vi "MasterAcquisitionFile_IOS_Test.vi"() -> ()   [LabVIEW 2020]
uses:
  <vilib>/vision/driver/IMAQdx.llb/IMAQdx Camera Control Mode.ctl
  <vilib>/vision/driver/IMAQdx.llb/IMAQdx Acquisition Mode.ctl
  <vilib>/userDefined/High Color/IMAQdx.ctl
  <vilib>/vision/driver/IMAQdx.llb/IMAQdx Buffer Number Mode.ctl
  <vilib>/DAQmx/write.llb/DAQmx Write (Digital 1D Wfm NChan NSamp).vi
  <vilib>/DAQmx/read.llb/DAQmx Read (Analog 1D Wfm NChan NSamp).vi
  <vilib>/Waveform/DWDTOps.llb/DWDT Digital to Boolean Array.vi
  <vilib>/DAQmx/create/channels.llb/DAQmx Create Channel (CO-Pulse Generation-Frequency).vi
  <vilib>/DAQmx/configure/timing.llb/DAQmx Timing (Implicit).vi
  <vilib>/DAQmx/create/channels.llb/DAQmx Create Channel (AI-Voltage-Basic).vi
  <vilib>/DAQmx/configure/timing.llb/DAQmx Timing (Sample Clock).vi
  <vilib>/DAQmx/configure/trigger.llb/DAQmx Start Trigger (Digital Edge).vi
  <vilib>/DAQmx/create/channels.llb/DAQmx Create Channel (DO-Digital Output).vi
  <vilib>/Waveform/DWDTOps.llb/DWDT Boolean Array to Digital.vi
  <vilib>/Waveform/DWDTOps.llb/DWDT Uncompress Digital.vi
  <vilib>/DAQmx/miscellaneous.llb/DAQmx Fill In Error Info.vi
  <vilib>/vision/driver/NI_Vision_Acquisition_Software.lvlib
  <resource>/objmgr/imaqdx.rc
  <resource>/objmgr/daqmx.rc
panel:
  out "LED":bool
  out "Auditory":bool
  out "RPad":bool
  out "LPad":bool
  out "Finished":bool
  in  "Generate Stimuli":bool=TRUE
  in  "Sol Stim Parameters":cluster{"Fs":dbl, "Samples":dbl}
  in  "LED Stim Parameters":cluster{"Fs":dbl, "Samples":dbl}
  in  "Sol Duty Cycle (%)":dbl=10.0
  in  "Sol Freq":dbl=1.0
  in  "Sol Dur (s)":dbl=1.0
  in  "LED Duty Cycle (%)":dbl=10.0
  in  "LED Freq":dbl=10.0
  in  "LED Dur (s)":dbl=2.0
  out "Stimulus Order":digitalwaveform[](graph)=[{"t0"=timestamp(0 s since 1904-01-01), "dt"=5e-05, "Y"={"transitions"=[], "data"=array18001000x1[18001000 elements]}}, {"t0"=timestamp(0 s since 1904-01-01), "dt"=5e-05, "Y"={"transitions"=[], "data"=array18001000x1[18001000 elements]}}, {"t0"=timestamp(0 s since 1904-01-01), "dt"=5e-05, "Y"={"transitions"=[], "data"=array18001000x1[18001000 elements]}}, {"t0"=timestamp(0 s since 1904-01-01), "dt"=5e-05, "Y"={"transitions"=[], "data"=array18001000x1[18001000 elements]}}]
  out "Solenoid Stim":digitalwaveform(graph)={"t0"=timestamp(0 s since 1904-01-01), "dt"=5e-05, "Y"={"transitions"=[], "data"=array20000x1[20000 elements]}}
  in  "Trial Offset (s)":dbl=15.0
  in  "Interstim (s)":dbl=30.0
  in  "Right Pad":dbl=1.0
  in  "Left Pad":dbl=1.0
  in  "Auditory":dbl=1.0
  in  "LED":dbl
  out "?":T1(plugin-control)
  out "?":T1(plugin-control)
  out "?":T1(plugin-control)
  out "?":T1(plugin-control)
  in  "stop":bool
  out "CBV Cam":bool=TRUE
  out "Pupil Cam":bool=TRUE
  out "Whisk Cam":bool=TRUE
  out "Web Cam":bool=TRUE
  out "Analog":bool=TRUE
  out "Web Cam Fs":dbl(knob)=30.0 scale=0.0..200.0
  out "CBV Cam Fs":dbl(knob)=30.019685039370078 scale=0.0..200.0
  out "Whisk Cam Fs":dbl(knob)=149.92503748125938 scale=0.0..200.0
  out "Last Whisk\nBuffer 2":u32=160
  out "Pupil Cam Fs":dbl(knob)=30.0 scale=0.0..200.0
  out "Dropped 2":u32(slide) caption="Pupil Cam" scale=0.0..99.0
  in  "Exposure Time (microsec)":string="10000"
  out "Dev1 Samples":i32=107434
  in  "Dev1 Analog Channels":string[](array[string])=["Cortical_LH", "Force_Sensor", "LPadSol", "RPadSol", "AudSol", "Hippocampus", "EMG", "Cortical_RH", "OptoLED"]
  in  "Analog Acquisition":cluster{"Analog Fs":u16}={"Analog Fs"=20000} {"Analog Fs" format="%0.0f"}
  in  "Sampling Rates":T2={"CBV Cam Fs"=30, "Whisk Cam Fs"=150, "Web Cam Fs"=15, "Pupil Cam Fs"=30}
  out "Notes Size":i32=8
  out "Notes Reversed":string[](array[string])=["Experimenter", "Animal ID", "Hemisphere", "Solenoid PSI", "Isoflurane time", "Session ID", "Amplifier Gain", "LED power (mW)"]
  out "Notes Array":string[](array[string])=["LED power (mW)", "Amplifier Gain", "Session ID", "Isoflurane time", "Solenoid PSI", "Hemisphere", "Animal ID", "Experimenter"]
  in  "Notes:":T3={"Experimenter"="Kevin", "Animal ID"="T220", "Hemisphere"="Both", "Solenoid PSI"="10", "Isoflurane time"="1000", "Session ID"="Imaging Session One", "Amplifier Gain"="10000", "LED power (mW)"="10"}
  in  "Target Path":path=path "D:/T220/Imaging Session One - 17 May 2021" caption="Final Save Location"
  out "Dropped":u32(slide) caption="Whisk Cam" scale=0.0..999.0
  out "Filename":string="210517_10_15_02"
  out "CBV Camera":bool
  out "Time Elapsed (Min)":cluster{dbl, dbl}(slide)={15.0, 0.08920117000000001} scale=0.0..15.0 scale format="%#_2g"
  in  "Time (min)":dbl(knob)=15.0 min=0.5 max=20.0 step=0.5 scale=0.0..20.0 scale format="%#_2g"
  in  "Temp Path":path=path "D:/LabVIEW Streamed Data" caption="Temporary Path for Streamed Data"
  out "Last CBV\nBuffer":i32=160
  out "Last Whisk\nBuffer":u32=804
  # "Dropped Frames"
  # "Stimuli"
  # "LPAD"
  # "RPAD"
  # "AUD"
  # "LED"
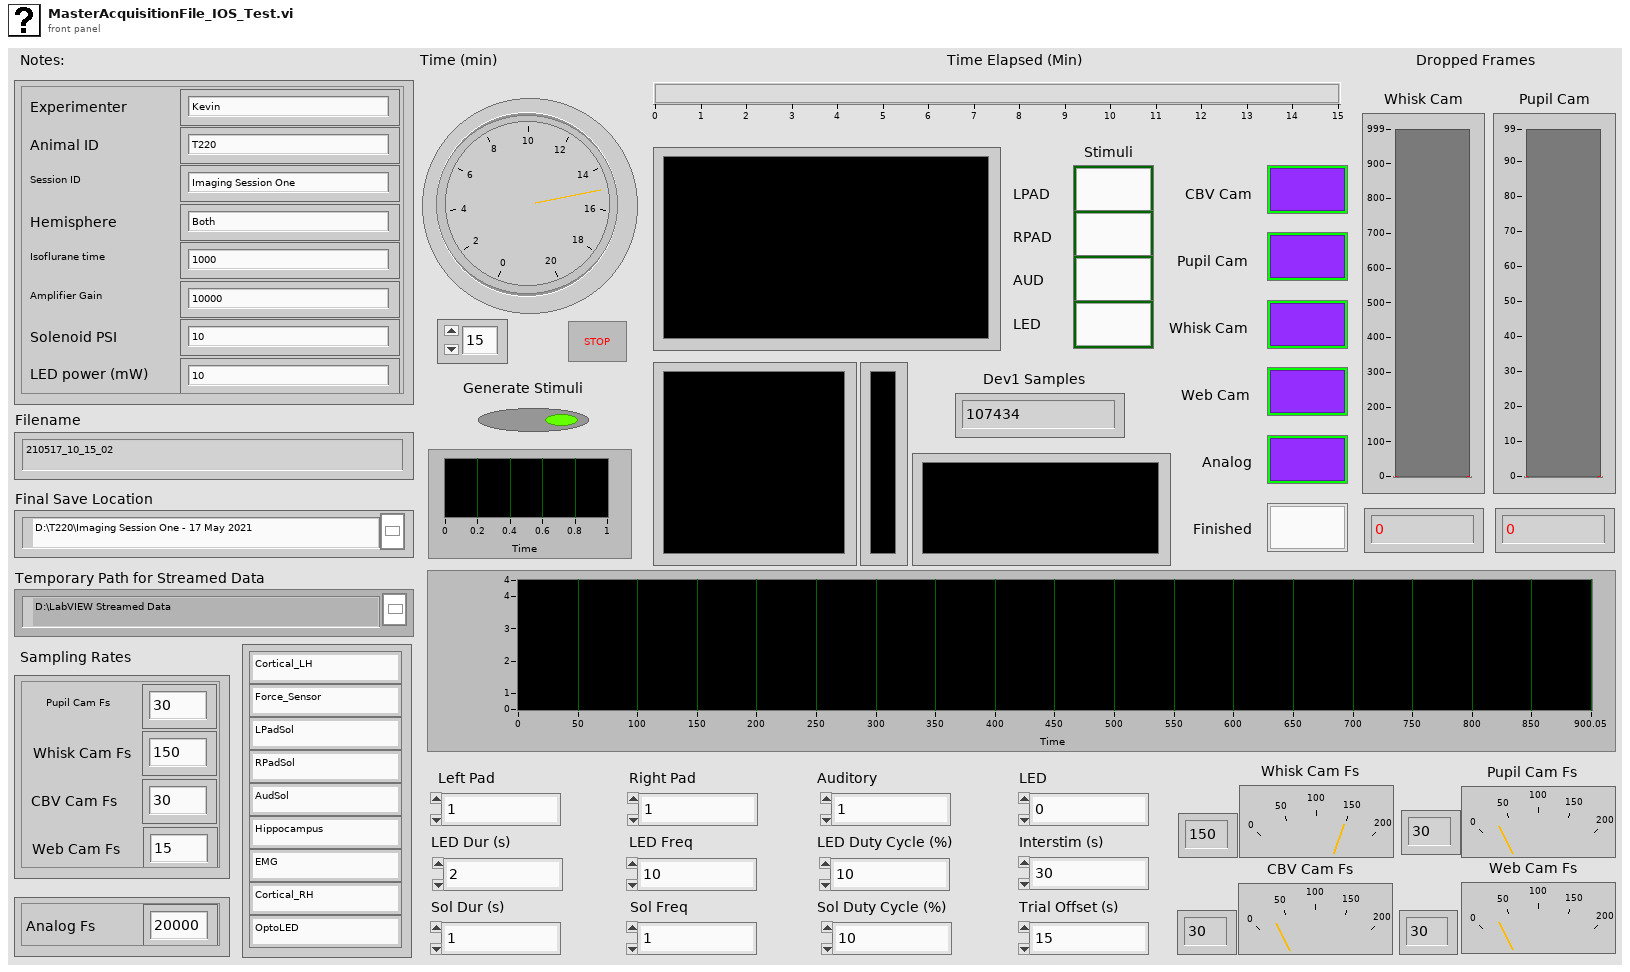
[diagram p1: front panel]
types:
  T1 = typedef "IMAQ Image.ctl" = refnum<image>
  T2 = cluster{"CBV Cam Fs":u16, "Whisk Cam Fs":u16, "Web Cam Fs":u16, "Pupil Cam Fs":u16}
  T3 = cluster{"Experimenter":string, "Animal ID":string, "Hemisphere":string, "Solenoid PSI":string, "Isoflurane time":string, "Session ID":string, "Amplifier Gain":string, "LED power (mW)":string}
  T4 = typedef "IMAQdx.ctl" = refnum<k21>
  T5 = enum16{"open", "replace", "create", "open or create", "replace or create", "replace or create with confirmation"}
  T6 = typedef "Image Type" = u32
  T7 = typedef "NI_Vision_Acquisition_Software.lvlib/IMAQdx Acquisition Mode.ctl" = enum32{"One Shot", "Continuous"}
  T8 = typedef "NI_Vision_Acquisition_Software.lvlib/IMAQdx Camera Control Mode.ctl" = enum32{"Controller", "Listener"}
  T9 = enum16{"open", "open or create", "create or replace", "create", "open (read-only)"}
  T10 = typedef "IMAQ AVI2 Refnum.ctl" = refnum<k20>
  T11 = enum16{"big-endian, network order", "native, host order", "little-endian"}
  T12 = typedef "NI_Vision_Acquisition_Software.lvlib/IMAQdx Buffer Number Mode.ctl" = enum32{"Next", "Last", "Buffer Number", "Every", "Last New"}
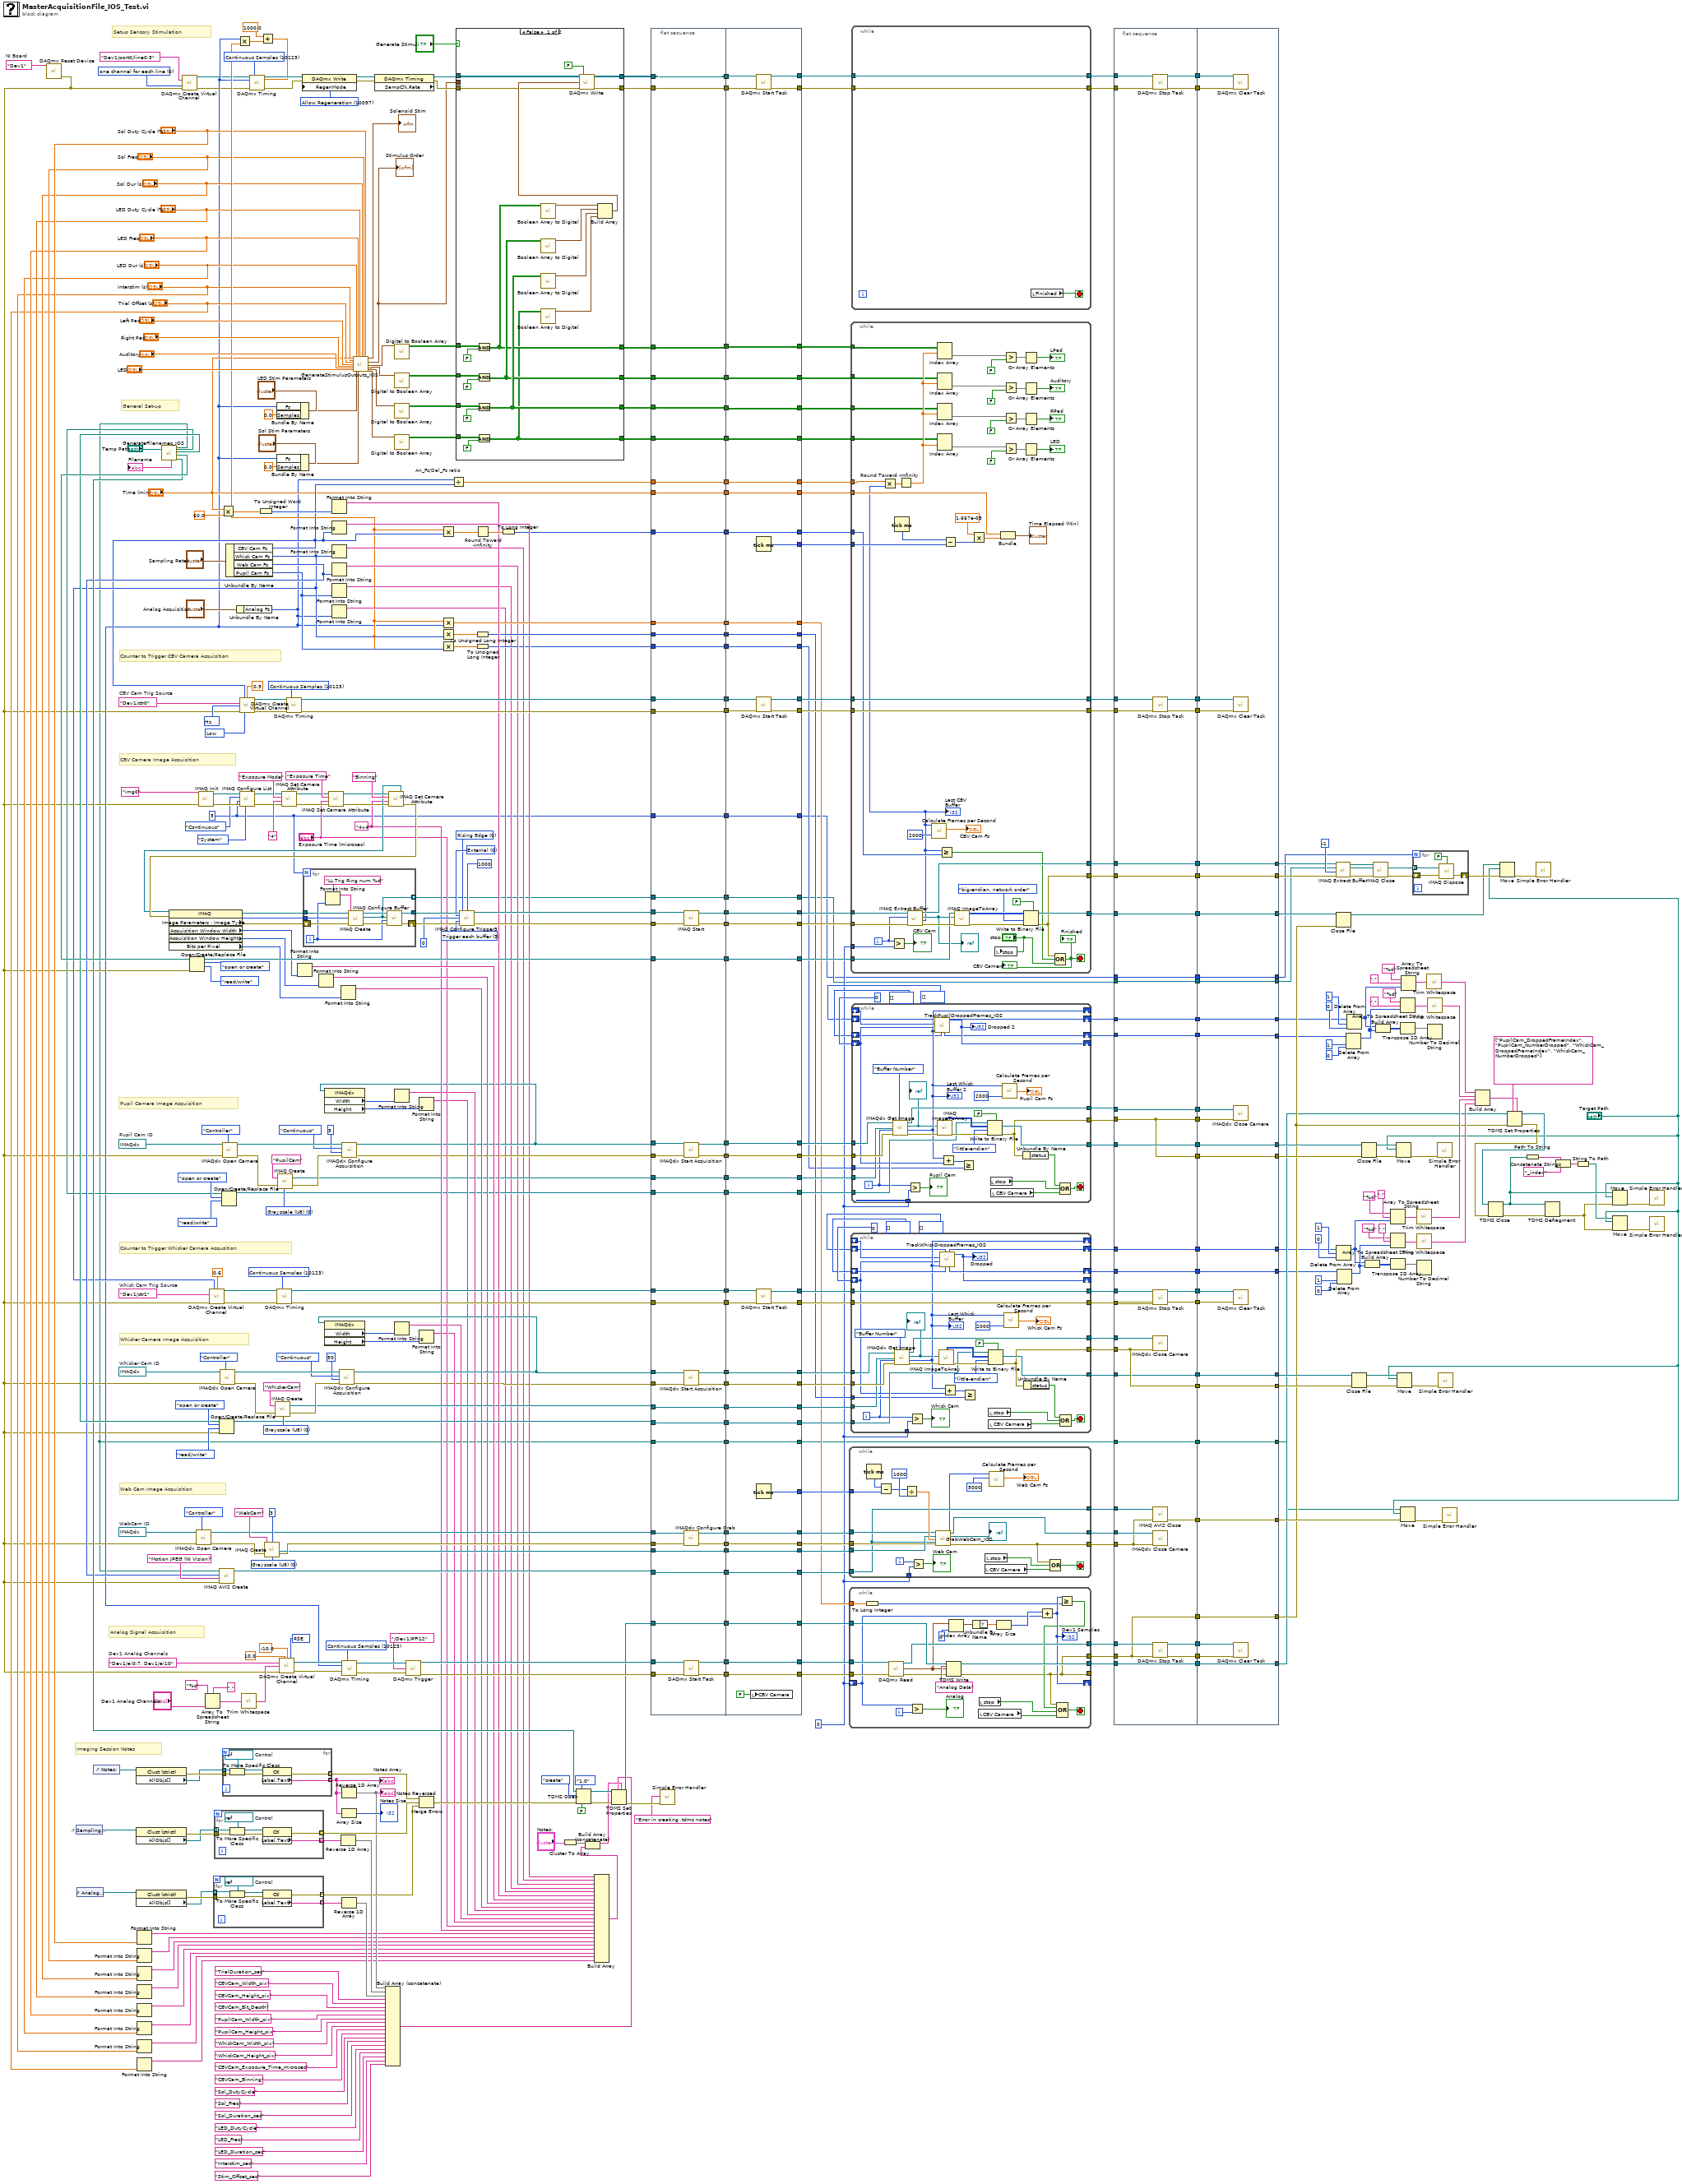
[diagram p0: block diagram]
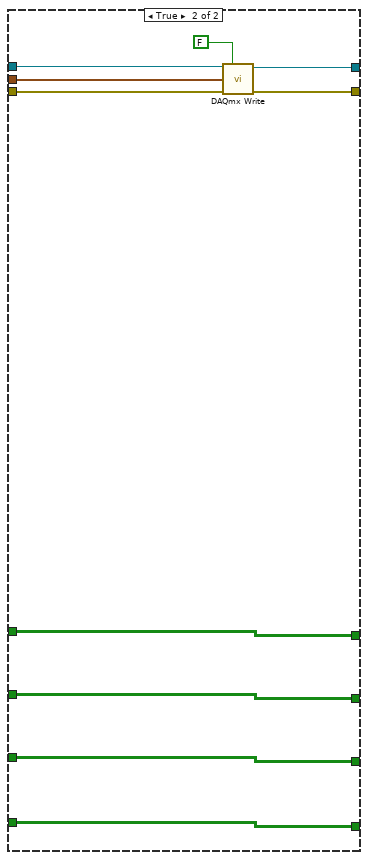
[diagram p2: hidden frame]
diagram:
  w109 = 10097 items=["Allow Regeneration"=10097, "Do Not Allow Regeneration"=10158] ("RegenMode")
  w110 = 10123 items=["Finite Samples"=10178, "Continuous Samples"=10123, "Hardware Timed Single Point"=12522] ("sample mode")
  w113 = 0 items=["one channel for each line", "one channel for all lines"] ("line grouping")
  w313 = tag "Dev1/ai0:7, Dev1/ai10"  # Dev1 Analog Channels
  w316 = T4 "cam0"  # WebCam ID
  w294 = T4 "cam1"  # Whisker Cam ID
  w470 = tag "Dev1/ctr1"  # Whisk Cam Trig Source
  w239 = T4 "cam2"  # Pupil Cam ID
  w75 = tag "Dev1/ctr0"  # CBV Cam Trig Source
  w242 = T6 0 items=["Grayscale (U8)", "Grayscale (I16)", "Grayscale (SGL)", "Complex (CSG)", "RGB (U32)", "HSL (U32)", "RGB (U64)", "Grayscale (U16)"] ("Image Type")
  w229 = "4x4" ("Attribute Value")
  w166 = 0
  w389 = 10123 items=["Finite Samples"=10178, "Continuous Samples"=10123, "Hardware Timed Single Point"=12522] ("sample mode")
  w392 = 10083 items=["default"=-1, "RSE"=10083, "NRSE"=10078, "Differential"=10106, "Pseudodifferential"=12529] ("input terminal configuration")
  w436 = T6 0 items=["Grayscale (U8)", "Grayscale (I16)", "Grayscale (SGL)", "Complex (CSG)", "RGB (U32)", "HSL (U32)", "RGB (U64)", "Grayscale (U16)"] ("Image Type")
  w452 = u32 0 items=["Rising Edge", "Falling Edge"] ("Trigger Polarity")
  w455 = u32 0 items=["External"=0, "RTSI"=1, "ISO In"=2, "Scaled Encoder"=5] ("Trigger Type")
  w446 = tag "Dev1"  # NI Board
  w447 = 10123 items=["Finite Samples"=10178, "Continuous Samples"=10123, "Hardware Timed Single Point"=12522] ("sample mode")
  w450 = 10373 items=["Hz"=10373] ("units")
  w451 = 10214 items=["High"=10192, "Low"=10214] ("idle state")
  w7 = u32 5 ("Number of Buffers")
  w453 = u32 3 items=["Disabled", "Trigger start of acquisition", "Trigger start of each buffer list", "Trigger each buffer", "Trigger each line (linescan)", "Trigger end of acquisition"] ("Action")
  w466 = 10123 items=["Finite Samples"=10178, "Continuous Samples"=10123, "Hardware Timed Single Point"=12522] ("sample mode")
  w473 = T6 0 items=["Grayscale (U8)", "Grayscale (I16)", "Grayscale (SGL)", "Complex (CSG)", "RGB (U32)", "HSL (U32)", "RGB (U64)", "Grayscale (U16)"] ("Image Type")
  # "General Set-up"
  # "Pupil Camera Image Acquisition"
  # "Whisker Camera Image Acquisition"
  # "Imaging Session Notes"
  # "Setup Sensory Stimulation"
  # "CBV Camera Image Acquisition"
  # "Counter to Trigger CBV Camera Acquisition"
  # "Counter to Trigger Whisker Camera Acqusition"
  # "Web Cam Image Acquisition"
  # "Analog Signal Acquisition"
  n1 = call <vilib>:"DAQmx Reset Device.vi"("device in"=w446) -> ("error out"=w67:errorcluster)  [unwired: 14 in]
  n2 = control-ref of="Sampling Rates"() -> (w322:refnum<vi>)
  n3 = control-ref of="Analog Acquisition"() -> (w321:refnum<vi>)
  n4 = control-ref of="Notes:"() -> (w343:refnum<vi>)
  n5 = property class="Clust (strict)"(reference=w343) -> (error out=w346:errorcluster, "AllObjs[]"=w258:refnum<vi>[])  [unwired: 1 in, 1 out]
  n6 = property class="Clust (strict)"(reference=w322) -> (error out=w341:errorcluster, "AllObjs[]"=w259:refnum<vi>[])  [unwired: 1 in, 1 out]
  n7 = property class="Clust (strict)"(reference=w321) -> (error out=w320:errorcluster, "AllObjs[]"=w257:refnum<vi>[])  [unwired: 1 in, 1 out]
  n8 = Format Into String("Sol Duty Cycle (%)") -> (resulting string=w143:string)  [unwired: 3 in, 1 out]
  n9 = Format Into String("Sol Freq") -> (resulting string=w142:string)  [unwired: 3 in, 1 out]
  n10 = Format Into String("Sol Dur (s)") -> (resulting string=w141:string)  [unwired: 3 in, 1 out]
  n11 = Format Into String("LED Duty Cycle (%)") -> (resulting string=w140:string)  [unwired: 3 in, 1 out]
  n12 = Format Into String("LED Freq") -> (resulting string=w139:string)  [unwired: 3 in, 1 out]
  n13 = Format Into String("LED Dur (s)") -> (resulting string=w138:string)  [unwired: 3 in, 1 out]
  n14 = Format Into String("Interstim (s)") -> (resulting string=w137:string)  [unwired: 3 in, 1 out]
  n15 = Format Into String("Trial Offset (s)") -> (resulting string=w136:string)  [unwired: 3 in, 1 out]
  n16 = call "GenerateFilenames_IOS.vi"("path"="Temp Path") -> ("TDMS Path"=w338:path, "Dalsa Path"=w443:path, "Basler Path"=w439:path, "WebCam Path"=w1:path, "Analog file name"=→"Filename":string, "Basler2 Path"=w238:path)  [unwired: 3 in, 2 out]
  n17 = call-poly <vilib>:"DAQmx Create Virtual Channel.vi"("lines"=tag "Dev1/port0/line0:3", "line grouping"=w113, "error in"=w67) -> ("task out"=w112:refnum<k21>, "error out"=w111:errorcluster)  [unwired: 11 in]
  n18 = Open/Create/Replace File(file path (use dialog)=w443, error in=w67, operation (0:open)=T5."open or create", access (0:read/write)=enum16{"read/write", "read-only", "write-only"}."read/write") -> (refnum out=w393:refnum<file>)  [unwired: 2 in, 2 out]
  n19 = call <vilib>:"IMAQdx Open Camera.vi"("Camera Control Mode"=IMAQdx_Camera_Control_Mode."Controller", "error in"=w67, "Session In"=w316) -> ("error out"=w432:errorcluster, "Session Out"=w430:T4)  [unwired: 7 in]
  n20 = call <vilib>:"IMAQ Init.vi"("error in (no error)"=w67, "Interface Name"="img0") -> ("error out"=w464:errorcluster, "IMAQ Session Out"=w465:refnum<k11>)  [unwired: 8 out]
  n21 = Array To Spreadsheet String(delimiter (Tab)=",", array="Dev1 Analog Channels", 3:"%s" ("format string")) -> (spreadsheet string=w310:string)
  n22 = for {
    tunnel: [w485] -> w318 mode=indexing
    tunnel: w320 -> [w484]
    tunnel: [w482] -> w319 mode=indexing
    tunnel: w257 -> [w481] mode=indexing
    w486 = refnum<vi> refnum  # Control
    n23 = To More Specific Class(target class=w486, reference=w481, error in=w484) -> (specific class reference=w487:refnum<vi>, error out=w483:errorcluster)
    n24 = property class="Ctl"(reference=w487, error in=w483) -> (error out=w482:errorcluster, "Label.Text"=w485:string)  [unwired: 1 out]
  }
  n25 = for {
    tunnel: [w492] -> w342 mode=indexing
    tunnel: w341 -> [w491]
    tunnel: [w489] -> w328 mode=indexing
    tunnel: w259 -> [w488] mode=indexing
    w493 = refnum<vi> refnum  # Control
    n26 = To More Specific Class(target class=w493, reference=w488, error in=w491) -> (specific class reference=w494:refnum<vi>, error out=w490:errorcluster)
    n27 = property class="Ctl"(reference=w494, error in=w490) -> (error out=w489:errorcluster, "Label.Text"=w492:string)  [unwired: 1 out]
  }
  n28 = Open/Create/Replace File(file path (use dialog)=w439, error in=w67, operation (0:open)=T5."open or create", access (0:read/write)=enum16{"read/write", "read-only", "write-only"}."read/write") -> (refnum out=w409:refnum<file>)  [unwired: 2 in, 2 out]
  n29 = call <vilib>:"IMAQdx Open Camera.vi"("Camera Control Mode"=IMAQdx_Camera_Control_Mode."Controller", "error in"=w67, "Session In"=w294) -> ("error out"=w476:errorcluster, "Session Out"=w479:T4)  [unwired: 7 in]
  n30 = Multiply(x="Time (min)", y=60.0) -> (x*y=w153:dbl)
  n31 = Open/Create/Replace File(file path (use dialog)=w238, operation (0:open)=T5."open or create", access (0:read/write)=enum16{"read/write", "read-only", "write-only"}."read/write") -> (refnum out=w219:refnum<file>)  [unwired: 3 in, 2 out]
  n32 = call <vilib>:"IMAQdx Open Camera.vi"("Camera Control Mode"=IMAQdx_Camera_Control_Mode."Controller", "error in"=w67, "Session In"=w239) -> ("error out"=w245:errorcluster, "Session Out"=w248:T4)  [unwired: 7 in]
  n33 = for {
    tunnel: [w499] -> w345 mode=indexing
    tunnel: w346 -> [w498]
    tunnel: [w496] -> w329 mode=indexing
    tunnel: w258 -> [w495] mode=indexing
    w500 = refnum<vi> refnum  # Control
    n34 = To More Specific Class(target class=w500, reference=w495, error in=w498) -> (specific class reference=w501:refnum<vi>, error out=w497:errorcluster)
    n35 = property class="Ctl"(reference=w501, error in=w497) -> (error out=w496:errorcluster, "Label.Text"=w499:string)  [unwired: 1 out]
  }
  "Notes Array" <- w345
  n36 = Unbundle By Name("Sampling Rates") -> ("CBV Cam Fs"=w154:u16, "Whisk Cam Fs"=w208:u16, "Web Cam Fs"=w315:u16, "Pupil Cam Fs"=w202:u16)
  n37 = call-poly <vilib>:"DAQmx Create Virtual Channel.vi"("frequency"=w208, "duty cycle"=0.6, "counter"=w470, "error in"=w67) -> ("task out"=w468:refnum<k21>, "error out"=w467:errorcluster)  [unwired: 10 in]
  n38 = call "IMAQ AVI2 Create"("error in (no error)"=w67, "Codec"="Motion JPEG (NI Vision)", "Frames Per Second"=w315, "AVI Path"=w1) -> ("AVI Refnum"=w422:T10)  [unwired: 6 in, 1 out]
  n39 = Unbundle By Name("Analog Acquisition") -> ("Analog Fs"=w126:u16)
  n40 = Multiply(x=w126, y=w153) -> (x*y=w86:dbl)
  n41 = call-poly <vilib>:"DAQmx Create Virtual Channel.vi"("frequency"=w154, "duty cycle"=0.9, "counter"=w75, "units"=w450, "error in"=w67, "idle state"=w451) -> ("task out"=w449:refnum<k21>, "error out"=w448:errorcluster)  [unwired: 8 in]
  n42 = call <vilib>:"IMAQ Configure List.vi"("Memory Location"=enum16{"System", "Onboard"}."System", "error in (no error)"=w464, "Number of buffers"=w7, "Continuous?"=enum16{"One-Shot", "Continuous"}."Continuous" ("Continuous ?"), "IMAQ Session In"=w465) -> ("error out"=w272:errorcluster, "IMAQ Session Out"=w268:refnum<k11>)  [unwired: 1 in, 4 out]
  n43 = call <vilib>:"Trim Whitespace.vi"("string"=w310) -> ("trimmed string"=w309:string)  [unwired: 1 in]
  n44 = To Unsigned Word Integer(number=w153) -> (unsigned 16bit integer=w305:u16)
  n45 = Add(x=1000.0, y=w86) -> (x+y=w84:dbl)
  n46 = call-poly <vilib>:"DAQmx Timing.vi"("task/channels in"=w112, "sample mode"=w110, "samples per channel"=w84, "rate"=w126, "error in"=w111) -> ("task out"=w106:refnum<k21>, "error out"=w105:errorcluster)  [unwired: 9 in]
  n47 = call "IMAQ Create"("Border Size"=3, "Image Name"="WebCam", "Image Type"=w436, "error in (no error)"=w432) -> ("New Image"=w429:T1, "error out"=w431:errorcluster)  [unwired: 1 in]
  n48 = call "IMAQ Create"("Image Name"="WhiskerCam", "Image Type"=w473, "error in (no error)"=w476) -> ("New Image"=w292:T1, "error out"=w474:errorcluster)  [unwired: 2 in]
  n49 = Bundle By Name(cluster="LED Stim Parameters", "Fs"=w126, "Samples"=0.0) -> (w159:cluster{"Fs":dbl, "Samples":dbl})
  n50 = Bundle By Name(cluster="Sol Stim Parameters", "Fs"=w126, "Samples"=0.0) -> (w160:cluster{"Fs":dbl, "Samples":dbl})
  n51 = call-poly <vilib>:"DAQmx Timing.vi"("task/channels in"=w468, "sample mode"=w466, "error in"=w467) -> ("task out"=w375:refnum<k21>, "error out"=w373:errorcluster)  [unwired: 11 in]
  n52 = call "IMAQ Create"("Image Name"="PupilCam", "Image Type"=w242, "error in (no error)"=w245) -> ("New Image"=w211:T1, "error out"=w243:errorcluster)  [unwired: 2 in]
  n53 = call-poly <vilib>:"DAQmx Create Virtual Channel.vi"("maximum value"=10.0, "minimum value"=-10.0, "input terminal configuration"=w392, "physical channels"=w313, "name to assign"=w309, "error in"=w67) -> ("task out"=w391:refnum<k21>, "error out"=w390:errorcluster)  [unwired: 8 in]
  n54 = call <vilib>:"IMAQ Set Camera Attribute.vi"("error in (no error)"=w272, "Attribute Value"="4", "Camera Attribute"="Exposure Mode", "IMAQ Session In"=w268) -> ("error out"=w271:errorcluster, "IMAQ Session Out"=w267:refnum<k11>)  [unwired: 4 in]
  n55 = call-poly <vilib>:"DAQmx Timing.vi"("task/channels in"=w449, "sample mode"=w447, "error in"=w448) -> ("task out"=w379:refnum<k21>, "error out"=w377:errorcluster)  [unwired: 11 in]
  n56 = property class="DAQmx Write"(reference=w106, error in=w105, "RegenMode"=w109) -> (reference out=w107:refnum<k21>, error out=w108:errorcluster)
  n57 = call <vilib>:"IMAQ Set Camera Attribute.vi"("error in (no error)"=w271, "Attribute Value"="Exposure Time (microsec)", "Camera Attribute"="Exposure Time", "IMAQ Session In"=w267) -> ("error out"=w270:errorcluster, "IMAQ Session Out"=w266:refnum<k11>)  [unwired: 4 in]
  n58 = Format Into String(w305) -> (resulting string=w307:string)  [unwired: 3 in, 1 out]
  n59 = Format Into String(w154) -> (resulting string=w206:string)  [unwired: 3 in, 1 out]
  n60 = Format Into String(w208) -> (resulting string=w205:string)  [unwired: 3 in, 1 out]
  n61 = Format Into String(w315) -> (resulting string=w204:string)  [unwired: 3 in, 1 out]
  n62 = Format Into String(w202) -> (resulting string=w172:string)  [unwired: 3 in, 1 out]
  n63 = Format Into String(w126) -> (resulting string=w171:string)  [unwired: 3 in, 1 out]
  n64 = call <vilib>:"IMAQdx Configure Acquisition.vi"("error in"=w474, "Number of Buffers"=u32 50, "Continuous?"=IMAQdx_Acquisition_Mode."Continuous", "Session In"=w479) -> ("error out"=w179:errorcluster, "Session Out"=w293:T4)  [unwired: 6 in]
  n65 = property class="IMAQdx"(reference=w293) -> ("Width"=w304:u32, "Height"=w303:u32)  [unwired: 1 in, 2 out]
  n66 = Reverse 1D Array(array=w342) -> (reversed array=w332:string[])
  n67 = Reverse 1D Array(array=w345) -> (reversed array=w256:string[])
  "Notes Reversed" <- w256
  n68 = Array Size(array=w345) -> (size(s)=→"Notes Size":i32)
  n69 = Reverse 1D Array(array=w318) -> (reversed array=w317:string[])
  n70 = call <vilib>:"IMAQdx Configure Acquisition.vi"("error in"=w243, "Number of Buffers"=u32 5, "Continuous?"=IMAQdx_Acquisition_Mode."Continuous", "Session In"=w248) -> ("error out"=w221:errorcluster, "Session Out"=w212:T4)  [unwired: 6 in]
  n71 = property class="IMAQdx"(reference=w212) -> ("Width"=w237:u32, "Height"=w236:u32)  [unwired: 1 in, 2 out]
  n72 = call-poly <vilib>:"DAQmx Timing.vi"("task/channels in"=w391, "sample mode"=w389, "rate"=w126, "error in"=w390) -> ("task out"=w255:refnum<k21>, "error out"=w388:errorcluster)  [unwired: 10 in]
  n73 = call "GenerateStimulusOutputs_IOS.vi"("Trial duration (min)"="Time (min)", "Rest duration(s)"="Interstim (s)", "trial offset (s)"="Trial Offset (s)", "Left Pad"="Left Pad", "Right Pad"="Right Pad", "Auditory"="Auditory", "LED"="LED", "LED Stim Duration (s)"="LED Dur (s)", "LED Stim Parameters"=w159, "LED Frequency"="LED Freq", "Sol Stim Parameters"=w160, "LED duty cycle (%)"="LED Duty Cycle (%)", "Sol Stim Duration (s)"="Sol Dur (s)", "Sol Frequency"="Sol Freq", "Sol Duty Cycle (%)"="Sol Duty Cycle (%)") -> ("Solenoid Stim Waveforms"=→"Solenoid Stim":digitalwaveform, "Stimulus Digital Outputs"=w87:digitalwaveform[], "Left Pad Out"=w117:digitalwaveform, "Auditory Out"=w116:digitalwaveform, "Right Pad Out"=w115:digitalwaveform, "LED Out"=w114:digitalwaveform)  [unwired: 7 in]
  "Stimulus Order" <- w87
  n74 = property class="DAQmx Timing" props=["SampClk.Rate"](reference=w107, error in=w108) -> (reference out=w103:refnum<k21>, error out=w102:errorcluster)  [unwired: 1 out]
  n75 = Build Array (concatenate)(w256, w332, w317, "TrialDuration_sec", "CBVCam_Width_pix", "CBVCam_Height_pix", "CBVCam_Bit_Depth", "PupilCam_Width_pix", "PupilCam_Height_pix", "WhiskCam_Width_pix", "WhiskCam_Height_pix", "CBVCam_Exposure_Time_microsec" ("element"), "CBVCam_Binning" ("element"), "Sol_DutyCycle", "Sol_Freq", "Sol_Duration_sec", "LED_DutyCycle", "LED_Freq", "LED_Duration_sec", "Interstim_sec", "Stim_Offset_sec") -> (w250:string[])
  n76 = call <vilib>:"IMAQ Set Camera Attribute.vi"("error in (no error)"=w270, "Attribute Value"=w229, "Camera Attribute"="Binning", "IMAQ Session In"=w266) -> ("error out"=w269:errorcluster, "IMAQ Session Out"=w265:refnum<k11>)  [unwired: 4 in]
  n77 = property class="IMAQ"(reference=w265, error in=w269) -> (reference out=w279:refnum<k11>, error out=w278:errorcluster, "Image Parameters : Image Type"=w460:u32, "Acquisition Window Width"=w302:u32, "Acquisition Window Height"=w301:u32, "Bits per Pixel"=w300:u32)
  n78 = Format Into String(w302) -> (resulting string=w299:string)  [unwired: 3 in, 1 out]
  n79 = for {
    N: w7 -> [_]
    tunnel: [w511] -> w457
    tunnel: w460 -> [w509]
    shift-right: [w510] -> w456
    shift-left: w278 -> [w508]
    tunnel: [w503] -> w12 mode=indexing
    tunnel: w279 -> [w502]
    i -> [w504]
    n80 = Format Into String(format string="LL Trig Ring num %d", w504) -> (resulting string=w506:string)  [unwired: 2 in, 1 out]
    n81 = call "IMAQ Create"("Image Name"=w506, "Image Type"=w509, "error in (no error)"=w508) -> ("New Image"=w503:T1, "error out"=w507:errorcluster)  [unwired: 1 in, 1 out]
    n82 = call <vilib>:"IMAQ Configure Buffer.vi"("error in (no error)"=w507, "Buffer Number"=w504, "Image In"=w503, "IMAQ Session In"=w502) -> ("error out"=w510:errorcluster, "IMAQ Session Out"=w511:refnum<k11>)  [unwired: 2 in, 4 out]
  }
  n83 = Format Into String(w301) -> (resulting string=w252:string)  [unwired: 3 in, 1 out]
  n84 = Format Into String(w300) -> (resulting string=w298:string)  [unwired: 3 in, 1 out]
  n85 = Format Into String(w237) -> (resulting string=w224:string)  [unwired: 3 in, 1 out]
  n86 = Format Into String(w304) -> (resulting string=w226:string)  [unwired: 3 in, 1 out]
  n87 = call-poly <vilib>:"Digital to Boolean Array.vi"("digital waveform"=w117) -> ("boolean array"=w95:bool[][])  [unwired: 9 in, 1 out]
  n88 = call-poly <vilib>:"Digital to Boolean Array.vi"("digital waveform"=w116) -> ("boolean array"=w94:bool[][])  [unwired: 9 in, 1 out]
  n89 = call-poly <vilib>:"Digital to Boolean Array.vi"("digital waveform"=w115) -> ("boolean array"=w93:bool[][])  [unwired: 9 in, 1 out]
  n90 = call-poly <vilib>:"Digital to Boolean Array.vi"("digital waveform"=w114) -> ("boolean array"=w92:bool[][])  [unwired: 9 in, 1 out]
  n91 = call-poly <vilib>:"DAQmx Trigger.vi"("task/channels in"=w255, "source"=tag "/Dev1/PFI12", "error in"=w388) -> ("task out"=w387:refnum<k21>, "error out"=w386:errorcluster)  [unwired: 11 in]
  n92 = Format Into String(w236) -> (resulting string=w225:string)  [unwired: 3 in, 1 out]
  n93 = Format Into String(w303) -> (resulting string=w227:string)  [unwired: 3 in, 1 out]
  n94 = Merge Errors(w329, w328, w319) -> (w327:errorcluster)
  n95 = Multiply(x=w153, y=w154) -> (x*y=w441:dbl)
  n96 = Multiply(x=w153, y=w126) -> (x*y=w283:dbl)
  n97 = Multiply(x=w208, y=w153) -> (x*y=w253:dbl)
  n98 = Multiply(x=w202, y=w153) -> (x*y=w207:dbl)
  n99 = Divide "An_Fs/Dal_Fs ratio"(x=w126, y=w154) -> (x/y=w70:dbl)
  n100 = case shown="False" "Generate Stimuli" {
    tunnel: w103 -> [w522 w543]
    tunnel: w102 -> [w521 w542]
    tunnel: [w519 w541] -> w100
    tunnel: [w520 w540] -> w98
    tunnel: w95 -> [w530 w539]
    tunnel: w94 -> [w531 w538]
    tunnel: w93 -> [w532 w537]
    tunnel: w92 -> [w533 w536]
    tunnel: [w514 w539] -> w91
    tunnel: [w515 w538] -> w90
    tunnel: [w516 w537] -> w89
    tunnel: [w512 w536] -> w88
    tunnel: w87 -> [_ w535]
    frame False {
      n101 = Compound Arithmetic op=AND(w530, FALSE) -> (w514:bool[][])
      n102 = Compound Arithmetic op=AND(w531, FALSE) -> (w515:bool[][])
      n103 = Compound Arithmetic op=AND(w532, FALSE) -> (w516:bool[][])
      n104 = Compound Arithmetic op=AND(w533, FALSE) -> (w512:bool[][])
      n105 = call-poly <vilib>:"Boolean Array to Digital.vi"("boolean array"=w514) -> ("digital waveform"=w524:digitalwaveform)  [unwired: 9 in, 1 out]
      n106 = call-poly <vilib>:"Boolean Array to Digital.vi"("boolean array"=w515) -> ("digital waveform"=w518:digitalwaveform)  [unwired: 9 in, 1 out]
      n107 = call-poly <vilib>:"Boolean Array to Digital.vi"("boolean array"=w516) -> ("digital waveform"=w517:digitalwaveform)  [unwired: 9 in, 1 out]
      n108 = call-poly <vilib>:"Boolean Array to Digital.vi"("boolean array"=w512) -> ("digital waveform"=w513:digitalwaveform)  [unwired: 9 in, 1 out]
      n109 = Build Array(w524, w518, w517, w513) -> (w523:digitalwaveform[])
      n110 = call-poly <vilib>:"DAQmx Write.vi"("task/channels in"=w522, "auto start"=FALSE, "data"=w523, "error in"=w521) -> ("task out"=w519:refnum<k21>, "error out"=w520:errorcluster)  [unwired: 9 in, 1 out]
    }
    frame True {
      n111 = call-poly <vilib>:"DAQmx Write.vi"("task/channels in"=w543, "auto start"=FALSE, "data"=w535, "error in"=w542) -> ("task out"=w541:refnum<k21>, "error out"=w540:errorcluster)  [unwired: 9 in, 1 out]
    }
  }
  n112 = call <vilib>:"IMAQ Configure Trigger3.vi"("IMAQ Session In"=w457, "Polarity"=w452, "Frame timeout (ms)"=u32 1000 ("Frame Timeout (ms)"), "Type"=w455, "Line Number"=u32 0 ("Trigger Line Number"), "Action"=w453, "error in (no error)"=w456) -> ("IMAQ Session Out"=w408:refnum<k11>, "error out"=w407:errorcluster)  [unwired: 2 in, 5 out]
  n113 = To Unsigned Long Integer(number=w253) -> (unsigned 32bit integer=w281:u32)
  n114 = To Unsigned Long Integer(number=w207) -> (unsigned 32bit integer=w203:u32)
  n115 = Round Toward -Infinity(1:w441) -> (0:w440:dbl)
  n116 = To Long Integer(number=w440) -> (32bit integer=w180:i32)
  n117 = Cluster To Array(cluster="Notes:") -> (array=w339:string[])
  n118 = TDMS Open(6:FALSE ("disable buffering? (T)"), 7:enum16{"1.0", "2.0"}."1.0" ("file format version (2.0)"), 8:w327, 10:T9."create" ("operation (0:open)"), 11:w338) -> (0:w333:errorcluster, 3:w334:refnum<k34>)  [unwired: 2 in]
  n119 = Build Array(w206, w205, w204, w172, w171, w307, w299, w252, w298, w224, w225, w226, w227, "Exposure Time (microsec)", w229, w143, w142, w141, w140, w139, w138, w137, w136) -> (w314:string[])
  n120 = Build Array (concatenate)(w339, w314) -> (w331:string[])
  n121 = TDMS Set Properties(5:w331, 7:w250, 8:w333, 11:w334) -> (0:w326:errorcluster, 3:w330:refnum<k34>)  [unwired: 2 in, 2 out]
  n122 = flat-sequence {
    tunnel: w431 -> [w590]
    tunnel: w430 -> [w589]
    tunnel: w429 -> [w588]
    tunnel: [w588] -> w428
    tunnel: [w587] -> w426
    tunnel: [w586] -> w424
    tunnel: w422 -> [w585]
    tunnel: [w585] -> w421
    tunnel: w293 -> [w584]
    tunnel: w179 -> [w583]
    tunnel: [w582] -> w416
    tunnel: [w581] -> w414
    tunnel: [w580] -> w412
    tunnel: w292 -> [w580]
    tunnel: [w579] -> w410
    tunnel: w409 -> [w579]
    tunnel: w408 -> [w578]
    tunnel: w407 -> [w577]
    tunnel: [w576] -> w405
    tunnel: [w575] -> w403
    tunnel: w180 -> [w574]
    tunnel: [w574] -> w399
    tunnel: "Time (min)" -> [w573]
    tunnel: [w573] -> w396
    tunnel: [w572] -> w394
    tunnel: w393 -> [w572]
    tunnel: w387 -> [w571]
    tunnel: w386 -> [w570]
    tunnel: [w569] -> w385
    tunnel: [w568] -> w384
    tunnel: [w567] -> w380
    tunnel: w330 -> [w567]
    tunnel: w379 -> [w566]
    tunnel: [w566] -> w378
    tunnel: w377 -> [w565]
    tunnel: [w565] -> w376
    tunnel: w375 -> [w564]
    tunnel: [w564] -> w374
    tunnel: w373 -> [w563]
    tunnel: [w563] -> w372
    tunnel: w283 -> [w562]
    tunnel: [w562] -> w282
    tunnel: w281 -> [w561]
    tunnel: [w561] -> w280
    tunnel: [w556] -> w223
    tunnel: w212 -> [w557]
    tunnel: [w554] -> w222
    tunnel: w221 -> [w555]
    tunnel: [w560] -> w220
    tunnel: w219 -> [w560]
    tunnel: w211 -> [w559]
    tunnel: [w559] -> w210
    tunnel: w203 -> [w558]
    tunnel: [w558] -> w201
    tunnel: [w553] -> w125
    tunnel: w91 -> [w553]
    tunnel: [w552] -> w124
    tunnel: w90 -> [w552]
    tunnel: [w551] -> w123
    tunnel: w89 -> [w551]
    tunnel: [w550] -> w122
    tunnel: w88 -> [w550]
    tunnel: [w549] -> w101
    tunnel: w100 -> [w549]
    tunnel: [w548] -> w99
    tunnel: w98 -> [w548]
    tunnel: w70 -> [w547]
    tunnel: [w547] -> w69
    tunnel: w12 -> [w546]
    tunnel: [w546] -> w15
    tunnel: w7 -> [w545]
    tunnel: [w545] -> w10
    tunnel: w1 -> [w544]
    tunnel: [w544] -> w2
    tunnel: [w636] -> w433
    tunnel: w428 -> [w635]
    tunnel: [w635] -> w427
    tunnel: w426 -> [w634]
    tunnel: [w634] -> w425
    tunnel: w424 -> [w633]
    tunnel: [w633] -> w423
    tunnel: w421 -> [w632]
    tunnel: [w632] -> w420
    tunnel: [w614] -> w419
    tunnel: [w613] -> w418
    tunnel: [w631] -> w417
    tunnel: w416 -> [w631]
    tunnel: [w630] -> w415
    tunnel: w414 -> [w630]
    tunnel: [w629] -> w413
    tunnel: w412 -> [w629]
    tunnel: [w628] -> w411
    tunnel: w410 -> [w628]
    tunnel: [w627] -> w406
    tunnel: w405 -> [w627]
    tunnel: [w626] -> w404
    tunnel: w403 -> [w626]
    tunnel: [w618] -> w402
    tunnel: [w617] -> w401
    tunnel: [w625] -> w400
    tunnel: w399 -> [w624]
    tunnel: [w624] -> w398
    tunnel: [w623] -> w397
    tunnel: w396 -> [w623]
    tunnel: [w622] -> w395
    tunnel: w394 -> [w622]
    tunnel: [w621] -> w382
    tunnel: w385 -> [w621]
    tunnel: [w620] -> w383
    tunnel: w384 -> [w620]
    tunnel: [w619] -> w169
    tunnel: w380 -> [w619]
    tunnel: w378 -> [w616]
    tunnel: w376 -> [w615]
    tunnel: w374 -> [w612]
    tunnel: w372 -> [w611]
    tunnel: w282 -> [w610]
    tunnel: [w610] -> w170
    tunnel: w280 -> [w609]
    tunnel: [w609] -> w200
    tunnel: w223 -> [w607]
    tunnel: w222 -> [w606]
    tunnel: w220 -> [w605]
    tunnel: [w607] -> w215
    tunnel: [w606] -> w214
    tunnel: [w605] -> w213
    tunnel: [w604] -> w209
    tunnel: w210 -> [w604]
    tunnel: [w603] -> w199
    tunnel: w201 -> [w603]
    tunnel: w125 -> [w599]
    tunnel: w124 -> [w602]
    tunnel: w123 -> [w601]
    tunnel: w122 -> [w600]
    tunnel: [w599] -> w121
    tunnel: [w602] -> w120
    tunnel: [w601] -> w119
    tunnel: [w600] -> w118
    tunnel: w101 -> [w598]
    tunnel: w99 -> [w597]
    tunnel: [w596] -> w97
    tunnel: [w595] -> w96
    tunnel: w69 -> [w594]
    tunnel: [w594] -> w68
    tunnel: w15 -> [w593]
    tunnel: [w593] -> w14
    tunnel: w10 -> [w592]
    tunnel: [w592] -> w9
    tunnel: [w591] -> w4
    tunnel: w2 -> [w591]
    frame #0 {
      n123 = call <vilib>:"IMAQ Start.vi"("error in (no error)"=w577, "IMAQ Session In"=w578) -> ("error out"=w575:errorcluster, "IMAQ Session Out"=w576:refnum<k11>)  [unwired: 8 out]
      n124 = call <vilib>:"IMAQdx Start Acquisition.vi"("error in"=w555, "Session In"=w557) -> ("error out"=w554:errorcluster, "Session Out"=w556:T4)  [unwired: 8 in]
      n125 = call <vilib>:"IMAQdx Start Acquisition.vi"("error in"=w583, "Session In"=w584) -> ("error out"=w581:errorcluster, "Session Out"=w582:T4)  [unwired: 8 in]
      n126 = call <vilib>:"IMAQdx Configure Grab.vi"("error in"=w590, "Session In"=w589) -> ("error out"=w586:errorcluster, "Session Out"=w587:T4)  [unwired: 8 in]
      n127 = call <vilib>:"DAQmx Start Task.vi"("task/channels in"=w571, "error in"=w570) -> ("task out"=w569:refnum<k21>, "error out"=w568:errorcluster)  [unwired: 12 in]
    }
    frame #1 {
      n128 = local write "CBV Camera"(FALSE ("Finished Acquiring")) -> ()
      n129 = call <vilib>:"DAQmx Start Task.vi"("task/channels in"=w598, "error in"=w597) -> ("task out"=w596:refnum<k21>, "error out"=w595:errorcluster)  [unwired: 12 in]
      n130 = Tick Count (ms)() -> (millisecond timer value=w625:u32)
      n131 = call <vilib>:"DAQmx Start Task.vi"("task/channels in"=w616, "error in"=w615) -> ("task out"=w618:refnum<k21>, "error out"=w617:errorcluster)  [unwired: 12 in]
      n132 = call <vilib>:"DAQmx Start Task.vi"("task/channels in"=w612, "error in"=w611) -> ("task out"=w614:refnum<k21>, "error out"=w613:errorcluster)  [unwired: 12 in]
      n133 = Tick Count (ms)() -> (millisecond timer value=w636:u32)
    }
  }
  n134 = call <vilib>:"Simple Error Handler.vi"("error source (\" \")"="Error in creating .tdms notes" ("error source (\" \")"), "error in (no error)"=w326) -> ()  [unwired: 3 in, 5 out]
  n135 = while {
    tunnel: w383 -> [w659]
    tunnel: w382 -> [w658]
    tunnel: w169 -> [w657]
    tunnel: [w656] -> w35
    tunnel: [w645] -> _
    tunnel: [w655] -> w66
    shift-right: [w649] -> _
    shift-left: w166 -> [w640]
    tunnel: [w645] -> w65
    tunnel: w170 -> [w643]
    i -> [w641]
    stop <- w646 stop-if-true
    n136 = To Long Integer(number=w643) -> (32bit integer=w644:i32)
    n137 = call-poly <vilib>:"DAQmx Read.vi"("task/channels in"=w658, "error in"=w659) -> ("task out"=w655:refnum<k21>, "data"=w637:waveform(dbl)[], "error out"=w648:errorcluster)  [unwired: 11 in]
    n138 = Greater?(x=w640, y=w641) -> (0:→"Analog":bool)
    n139 = TDMS Write(0:w657, 5:"Analog Data" ("group name in (Untitled)"), 9:w637, 11:w648) -> (4:w656:refnum<k34>, 15:w645:errorcluster)  [unwired: 2 in, 2 out]
    n140 = Index Array(array=w637, index=0) -> (element=w652:waveform(dbl))
    n141 = Unbundle By Name(w652) -> ("Y"=w651:dbl[])
    n142 = local read "CBV Camera"() -> (w639:bool)
    n143 = local read "stop"() -> (w638:bool)
    n144 = Array Size(array=w651) -> (size(s)=w650:i32)
    n145 = Add(x=w650, y=w640) -> (x+y=w649:i32)
    "Dev1 Samples" <- w649
    n146 = Greater Or Equal?(x=w649, y=w644) -> (x >= y?=w647:bool)
    n147 = Compound Arithmetic op=OR(w645, w647, w638, w639) -> (w646:bool)
  }
  n148 = while {
    tunnel: w433 -> [w676]
    tunnel: w427 -> [w674]
    tunnel: w425 -> [w673]
    tunnel: w423 -> [w672]
    tunnel: w420 -> [w670]
    tunnel: [w671] -> w57
    tunnel: [w662] -> w58
    tunnel: [w670] -> w56
    tunnel: w166 -> [w665]
    i -> [w666]
    stop <- w663 stop-if-true
    n149 = Tick Count (ms)() -> (millisecond timer value=w678:u32)
    n150 = Subtract(x=w678, y=w676) -> (x-y=w679:u32)
    n151 = Divide(x=w679, y=u32 1000) -> (x/y=w675:dbl)
    n152 = Greater?(x=w666, y=w665) -> (0:→"Web Cam":bool)
    n153 = call "GrabWebCam_IOS.vi"("Session In"=w673, "Image In"=w674, "Trial Time"=w675, "AVI Refnum"=w670, "error in"=w672) -> ("Session Out"=w671:T4, "WebCam Img Out"=→"?":T1, "Buffer Number Out"=w669:u32, "error out"=w662:errorcluster)  [unwired: 7 in]
    n154 = local read "CBV Camera"() -> (w664:bool)
    n155 = local read "stop"() -> (w661:bool)
    n156 = call <vilib>:"Calculate Frames per Second.vi"("Update Interval (ms)"=u32 5000, "Buffer Number"=w669) -> ("Processed Frames/s"=→"Web Cam Fs":dbl)  [unwired: 7 in, 2 out]
    n157 = Compound Arithmetic op=OR(w662, w661, w664) -> (w663:bool)
  }
  n158 = while {
    tunnel: w406 -> [w733]
    tunnel: w404 -> [w734]
    tunnel: [w716] -> w18
    tunnel: [w714] -> w21
    tunnel: [w728] -> w46
    tunnel: [w723] -> w79
    tunnel: w402 -> [w723]
    tunnel: [w722] -> w78
    tunnel: w401 -> [w722]
    tunnel: w400 -> [w721]
    tunnel: w398 -> [w720]
    tunnel: w397 -> [w719]
    tunnel: w395 -> [w713]
    tunnel: w166 -> [w708]
    tunnel: w121 -> [w692]
    tunnel: w120 -> [w693]
    tunnel: w119 -> [w687]
    tunnel: w118 -> [w684]
    tunnel: w68 -> [w681]
    i -> [w709]
    stop <- w703 stop-if-true
    n159 = Greater?(x=w709, y=w708) -> (0:→"CBV Cam":bool)
    n160 = Tick Count (ms)() -> (millisecond timer value=w726:u32)
    n161 = call <vilib>:"IMAQ Extract Buffer.vi"("error in (no error)"=w734, "Buffer to extract"=w709, "IMAQ Session In"=w733) -> ("error out"=w727:errorcluster, "Buffer Number"=w704:i32, "Image Out"=w706:T1, "IMAQ Session Out"=w714:refnum<k11>)  [unwired: 5 out]
    "Last CBV\nBuffer" <- w704
    "?" <- w706
    n162 = Multiply(x=w681, y=w704) -> (x*y=w705:dbl)
    n163 = Round Toward -Infinity(1:w705) -> (0:w698:dbl)
    n164 = call <vilib>:"Calculate Frames per Second.vi"("Update Interval (ms)"=u32 2000, "Buffer Number"=w704) -> ("Processed Frames/s"=→"CBV Cam Fs":dbl)  [unwired: 7 in, 2 out]
    n165 = Index Array(array=w692, index (row)=w698) -> (element=w691:bool[])  [unwired: 1 in]
    n166 = Index Array(array=w693, index (row)=w698) -> (element=w689:bool[])  [unwired: 1 in]
    n167 = Index Array(array=w687, index (row)=w698) -> (element=w686:bool[])  [unwired: 1 in]
    n168 = Index Array(array=w684, index (row)=w698) -> (element=w683:bool[])  [unwired: 1 in]
    n169 = Greater Or Equal?(x=w704, y=w720) -> (x >= y?=w712:bool)
    n170 = Subtract(x=w726, y=w721) -> (x-y=w725:u32)
    n171 = call "IMAQ ImageToArray"("error in (no error)"=w727, "Image"=w706) -> ("error out"=w732:errorcluster, "Image Pixels (I16)"=w731:i16[][])  [unwired: 2 in, 3 out]
    n172 = Multiply(x=w725, y=1.667e-05) -> (x*y=w724:dbl)
    n173 = local write "stop"("stop") -> ()
    n174 = Bundle("Time (min)"=w719, w724) -> (→"Time Elapsed (Min)":cluster{"Time (min)":dbl, dbl})  [unwired: 1 in]
    n175 = Greater?(x=w691, y=FALSE ("Boolean")) -> (0:w690:bool[])
    n176 = Greater?(x=w689, y=FALSE ("Boolean")) -> (0:w688:bool[])
    n177 = Greater?(x=w686, y=FALSE ("Boolean")) -> (0:w685:bool[])
    n178 = Greater?(x=w683, y=FALSE ("Boolean")) -> (0:w682:bool[])
    n179 = Or Array Elements(Boolean array=w690) -> (logical OR=→"LPad":bool)
    n180 = Or Array Elements(Boolean array=w688) -> (logical OR=→"Auditory":bool)
    n181 = Or Array Elements(Boolean array=w685) -> (logical OR=→"RPad":bool)
    n182 = Or Array Elements(Boolean array=w682) -> (logical OR=→"LED":bool)
    n183 = Write to Binary File(file (use dialog)=w713, data=w731, error in=w732, 5:FALSE ("prepend array or string size? (T)"), 9:T11."big-endian, network order" ("byte order (0:big-endian, network order)")) -> (refnum out=w728:refnum<file>, error out=w716:errorcluster)  [unwired: 1 in, 1 out]
    n184 = Compound Arithmetic op=OR(w716, w712, "stop") -> (w703:bool)
    "CBV Camera" <- w703
    "Finished" <- w703
  }
  n185 = while {
    tunnel: w419 -> [w761]
    tunnel: [w762] -> w61
    tunnel: w418 -> [w762]
    tunnel: [w761] -> w62
    tunnel: [w754] -> w52
    tunnel: [w755] -> w53
    tunnel: [w760] -> w48
    tunnel: w417 -> [w759]
    tunnel: w415 -> [w758]
    tunnel: w413 -> [w757]
    tunnel: w411 -> [w756]
    shift-right: [w745] -> _
    shift-left: _ -> [w743]
    shift-right: [w740] -> _
    shift-left: u32 0 ("New Lost") -> [w744]
    shift-right: [w741] -> w30
    shift-left: u32[] [] ("NewBuffNum") -> [w742]
    shift-right: [w747] -> w33
    shift-left: u32[] [] ("NewNumLost") -> [w746]
    tunnel: w200 -> [w752]
    tunnel: w166 -> [w748]
    i -> [w735]
    stop <- w751 stop-if-true
    n186 = call <vilib>:"IMAQdx Get Image.vi"("Buffer Number Mode (Next)"=IMAQdx_Buffer_Number_Mode."Buffer Number", "error in"=w758, "Buffer Number In"=w735, "Image In"=w757, "Session In"=w759) -> ("error out"=w768:errorcluster, "Buffer Number Out"=w745:u32, "Image Out"=w737:T1, "Session Out"=w754:T4)  [unwired: 3 in]
    "Last Whisk\nBuffer" <- w745
    "?" <- w737
    n187 = Greater?(x=w735, y=w748) -> (0:→"Whisk Cam":bool)
    n188 = call "IMAQ ImageToArray"("error in (no error)"=w768, "Image"=w737) -> ("error out"=w767:errorcluster, "Image Pixels (U8)"=w766:u8[][])  [unwired: 2 in, 3 out]
    n189 = call "TrackWhiskDroppedFrames_IOS.vi"("NumLost"=w746, "BuffNum"=w742, "Curr Buffer"=w745, "Prev Lost"=w744, "Prev Buffer"=w743) -> ("New Lost"=w740:u32, "NewNumLost"=w747:u32[], "NewBuffNum"=w741:u32[])  [unwired: 4 in]
    "Dropped" <- w740
    n190 = Add(x=w745, y=w744) -> (x+y=w753:u32)
    n191 = Greater Or Equal?(x=w753, y=w752) -> ()  [unwired: 1 out]
    n192 = Write to Binary File(file (use dialog)=w756, data=w766, error in=w767, 5:FALSE ("prepend array or string size? (T)"), 9:T11."little-endian" ("byte order (0:big-endian, network order)")) -> (refnum out=w760:refnum<file>, error out=w755:errorcluster)  [unwired: 1 in, 1 out]
    n193 = local read "stop"() -> (w739:bool)
    n194 = local read "CBV Camera"() -> (w738:bool)
    n195 = call <vilib>:"Calculate Frames per Second.vi"("Update Interval (ms)"=u32 2000, "Buffer Number"=w745) -> ("Processed Frames/s"=→"Whisk Cam Fs":dbl)  [unwired: 7 in, 2 out]
    n196 = Unbundle By Name(w755) -> ("status"=w736:bool)
    n197 = Compound Arithmetic op=OR(w736, w739, w738) -> (w751:bool)
  }
  n198 = while {
    tunnel: w97 -> [w770]
    tunnel: [w771] -> w82
    tunnel: w96 -> [w771]
    tunnel: [w770] -> w83
    stop <- w772 stop-if-true
    n199 = local read "Finished"() -> (w772:bool)
  }
  n200 = while {
    tunnel: [w787] -> w73
    tunnel: [w788] -> w72
    tunnel: [w797] -> w43
    tunnel: w215 -> [w796]
    tunnel: w214 -> [w795]
    tunnel: w209 -> [w794]
    tunnel: w213 -> [w793]
    shift-right: [w786] -> _
    shift-left: _ -> [w792]
    shift-right: [w791] -> _
    shift-left: u32 0 ("New Lost") -> [w785]
    shift-right: [w790] -> w24
    shift-left: u32[] [] ("NewBuffNum") -> [w781]
    shift-right: [w789] -> w27
    shift-left: u32[] [] ("NewNumLost") -> [w782]
    tunnel: w199 -> [w780]
    tunnel: w166 -> [w778]
    i -> [w773]
    stop <- w783 stop-if-true
    n201 = call <vilib>:"IMAQdx Get Image.vi"("Buffer Number Mode (Next)"=IMAQdx_Buffer_Number_Mode."Buffer Number", "error in"=w795, "Buffer Number In"=w773, "Image In"=w794, "Session In"=w796) -> ("error out"=w804:errorcluster, "Buffer Number Out"=w786:u32, "Image Out"=w775:T1, "Session Out"=w787:T4)  [unwired: 3 in]
    "Last Whisk\nBuffer 2" <- w786
    "?" <- w775
    n202 = Greater?(x=w773, y=w778) -> (0:→"Pupil Cam":bool)
    n203 = call "TrackPupilDroppedFrames_IOS.vi"("NumLost"=w782, "BuffNum"=w781, "Curr Buffer"=w786, "Prev Lost"=w785, "Prev Buffer"=w792) -> ("New Lost"=w791:u32, "NewNumLost"=w789:u32[], "NewBuffNum"=w790:u32[])  [unwired: 4 in]
    "Dropped 2" <- w791
    n204 = call "IMAQ ImageToArray"("error in (no error)"=w804, "Image"=w775) -> ("error out"=w803:errorcluster, "Image Pixels (U8)"=w802:u8[][])  [unwired: 2 in, 3 out]
    n205 = Add(x=w786, y=w785) -> (x+y=w784:u32)
    n206 = Greater Or Equal?(x=w784, y=w780) -> ()  [unwired: 1 out]
    n207 = Write to Binary File(file (use dialog)=w793, data=w802, error in=w803, 5:FALSE ("prepend array or string size? (T)"), 9:T11."little-endian" ("byte order (0:big-endian, network order)")) -> (refnum out=w797:refnum<file>, error out=w788:errorcluster)  [unwired: 1 in, 1 out]
    n208 = local read "stop"() -> (w777:bool)
    n209 = local read "CBV Camera"() -> (w776:bool)
    n210 = call <vilib>:"Calculate Frames per Second.vi"("Update Interval (ms)"=u32 2000, "Buffer Number"=w786) -> ("Processed Frames/s"=→"Pupil Cam Fs":dbl)  [unwired: 7 in, 2 out]
    n211 = Unbundle By Name(w788) -> ("status"=w774:bool)
    n212 = Compound Arithmetic op=OR(w774, w777, w776) -> (w783:bool)
  }
  n213 = flat-sequence {
    tunnel: w83 -> [w842]
    tunnel: w82 -> [w841]
    tunnel: [w840] -> w81
    tunnel: [w839] -> w80
    tunnel: w79 -> [w838]
    tunnel: w78 -> [w837]
    tunnel: [w836] -> w77
    tunnel: [w835] -> w76
    tunnel: [w834] -> w74
    tunnel: w73 -> [w834]
    tunnel: w72 -> [w817]
    tunnel: [w817] -> w71
    tunnel: w66 -> [w833]
    tunnel: w65 -> [w816]
    tunnel: [w832] -> w64
    tunnel: [w831] -> w63
    tunnel: w62 -> [w830]
    tunnel: w61 -> [w829]
    tunnel: [w828] -> _
    tunnel: [w827] -> _
    tunnel: [w828] -> w60
    tunnel: [w827] -> w59
    tunnel: w58 -> [w825]
    tunnel: w57 -> [w826]
    tunnel: w56 -> [w824]
    tunnel: [w823] -> w55
    tunnel: w53 -> [w821]
    tunnel: w52 -> [w822]
    tunnel: [w821] -> w50
    tunnel: [w820] -> w49
    tunnel: w48 -> [w820]
    tunnel: w46 -> [w819]
    tunnel: [w819] -> w45
    tunnel: w43 -> [w818]
    tunnel: [w818] -> w42
    tunnel: [w817] -> w39
    tunnel: [w816] -> w38
    tunnel: w35 -> [w815]
    tunnel: [w815] -> w36
    tunnel: w33 -> [w814]
    tunnel: [w814] -> w32
    tunnel: w30 -> [w813]
    tunnel: [w813] -> w29
    tunnel: w27 -> [w812]
    tunnel: [w812] -> w26
    tunnel: w24 -> [w811]
    tunnel: [w811] -> w23
    tunnel: w21 -> [w810]
    tunnel: [w810] -> w20
    tunnel: w18 -> [w809]
    tunnel: [w809] -> w17
    tunnel: w14 -> [w808]
    tunnel: [w808] -> w13
    tunnel: w9 -> [w807]
    tunnel: [w807] -> w8
    tunnel: w4 -> [w806]
    tunnel: [w806] -> w3
    tunnel: w81 -> [w869]
    tunnel: w80 -> [w868]
    tunnel: w77 -> [w867]
    tunnel: w76 -> [w866]
    tunnel: w74 -> [w865]
    tunnel: w71 -> [w864]
    tunnel: w64 -> [w863]
    tunnel: w63 -> [w862]
    tunnel: w60 -> [w861]
    tunnel: w59 -> [w860]
    tunnel: w55 -> [w859]
    tunnel: [w859] -> w54
    tunnel: [w858] -> w51
    tunnel: w50 -> [w858]
    tunnel: w49 -> [w857]
    tunnel: [w857] -> w47
    tunnel: w45 -> [w856]
    tunnel: [w856] -> w44
    tunnel: w42 -> [w855]
    tunnel: [w855] -> w41
    tunnel: [w854] -> w40
    tunnel: w39 -> [w854]
    tunnel: w38 -> [w853]
    tunnel: [w853] -> w37
    tunnel: w36 -> [w852]
    tunnel: [w852] -> w34
    tunnel: w32 -> [w851]
    tunnel: [w851] -> w31
    tunnel: [w850] -> w28
    tunnel: w29 -> [w850]
    tunnel: w26 -> [w849]
    tunnel: [w849] -> w25
    tunnel: w23 -> [w848]
    tunnel: [w848] -> w22
    tunnel: w20 -> [w847]
    tunnel: [w847] -> w19
    tunnel: w17 -> [w846]
    tunnel: [w846] -> w16
    tunnel: w13 -> [w845]
    tunnel: [w845] -> w11
    tunnel: w8 -> [w844]
    tunnel: [w844] -> w6
    tunnel: [w843] -> w5
    tunnel: w3 -> [w843]
    frame #0 {
      n214 = call <vilib>:"DAQmx Stop Task.vi"("task/channels in"=w842, "error in"=w841) -> ("task out"=w840:refnum<k21>, "error out"=w839:errorcluster)  [unwired: 12 in]
      n215 = call <vilib>:"DAQmx Stop Task.vi"("task/channels in"=w838, "error in"=w837) -> ("task out"=w836:refnum<k21>, "error out"=w835:errorcluster)  [unwired: 12 in]
      n216 = call <vilib>:"DAQmx Stop Task.vi"("task/channels in"=w830, "error in"=w829) -> ("task out"=w828:refnum<k21>, "error out"=w827:errorcluster)  [unwired: 12 in]
      n217 = call <vilib>:"IMAQdx Close Camera.vi"("error in"=w821, "Session In"=w822) -> ()  [unwired: 9 in, 1 out]
      n218 = call "IMAQ AVI2 Close"("error in (no error)"=w825, "AVI Refnum"=w824) -> ("error out"=w823:errorcluster)  [unwired: 9 in]
      n219 = call <vilib>:"IMAQdx Close Camera.vi"("error in"=w825, "Session In"=w826) -> ()  [unwired: 9 in, 1 out]
      n220 = call <vilib>:"DAQmx Stop Task.vi"("task/channels in"=w833, "error in"=w816) -> ("task out"=w832:refnum<k21>, "error out"=w831:errorcluster)  [unwired: 12 in]
    }
    frame #1 {
      n221 = call <vilib>:"DAQmx Clear Task.vi"("task in"=w869, "error in"=w868) -> ()  [unwired: 13 in, 1 out]
      n222 = call <vilib>:"DAQmx Clear Task.vi"("task in"=w867, "error in"=w866) -> ()  [unwired: 13 in, 1 out]
      n223 = call <vilib>:"IMAQdx Close Camera.vi"("error in"=w864, "Session In"=w865) -> ()  [unwired: 9 in, 1 out]
      n224 = call <vilib>:"DAQmx Clear Task.vi"("task in"=w861, "error in"=w860) -> ()  [unwired: 13 in, 1 out]
      n225 = call <vilib>:"DAQmx Clear Task.vi"("task in"=w863, "error in"=w862) -> ()  [unwired: 13 in, 1 out]
    }
  }
  n226 = call <vilib>:"IMAQ Extract Buffer.vi"("error in (no error)"=w16, "Buffer to extract"=-1, "IMAQ Session In"=w19) -> ("error out"=w462:errorcluster, "IMAQ Session Out"=w461:refnum<k11>)  [unwired: 7 out]
  n227 = Close File(refnum=w44, error in=w37) -> (path=w361:path)  [unwired: 1 out]
  n228 = Delete From Array(array=w28, length=1, index=0) -> (array with subset deleted=w261:u32[])  [unwired: 1 out]
  n229 = Delete From Array(array=w31, length=1, index=0) -> (array with subset deleted=w262:u32[])  [unwired: 1 out]
  n230 = Delete From Array(array=w25, length=1, index=0) -> (array with subset deleted=w186:u32[])  [unwired: 1 out]
  n231 = Delete From Array(array=w22, length=1, index=0) -> (array with subset deleted=w185:u32[])  [unwired: 1 out]
  n232 = Close File(refnum=w47, error in=w51) -> (path=w360:path, error out=w359:errorcluster)
  n233 = Close File(refnum=w41, error in=w40) -> (path=w182:path, error out=w181:errorcluster)
  n234 = Build Array(w261, w262) -> (w264:u32[][])
  n235 = call <vilib>:"IMAQ Close.vi"("error in (no error)"=w462, "IMAQ Session In"=w461) -> ("error out"=w463:errorcluster)  [unwired: 9 out]
  n236 = Build Array(w185, w186) -> (w188:u32[][])
  n237 = Array To Spreadsheet String(delimiter (Tab)=",", array=w262, 3:"%d" ("format string")) -> (spreadsheet string=w284:string)
  n238 = Transpose 2D Array(2D array=w264) -> (transposed array=w263:u32[][])
  n239 = Array To Spreadsheet String(delimiter (Tab)=",", array=w261, 3:"%d" ("format string")) -> (spreadsheet string=w285:string)
  n240 = Move(source path=w182, error in=w181, 10:"Target Path") -> (error out=w183:errorcluster)  [unwired: 2 in, 2 out]
  n241 = Move(source path=w360, error in=w359, 10:"Target Path") -> (error out=w357:errorcluster)  [unwired: 2 in, 2 out]
  n242 = Array To Spreadsheet String(delimiter (Tab)=",", array=w186, 3:"%d" ("format string")) -> (spreadsheet string=w189:string)
  n243 = Transpose 2D Array(2D array=w188) -> (transposed array=w187:u32[][])
  n244 = Move(source path=w5, error in=w54, 10:"Target Path") -> (error out=w356:errorcluster)  [unwired: 2 in, 2 out]
  n245 = Array To Spreadsheet String(delimiter (Tab)=",", array=w185, 3:"%d" ("format string")) -> (spreadsheet string=w190:string)
  n246 = for {
    N: w6 -> [_]
    tunnel: w11 -> [w873] mode=indexing
    shift-right: [w871] -> w363
    shift-left: w463 -> [w872]
    n247 = call "IMAQ Dispose"("All Images? (No)"=FALSE, "Image"=w873, "error in (no error)"=w872) -> ("error out"=w871:errorcluster)  [unwired: 3 out]
  }
  n248 = call <vilib>:"Trim Whitespace.vi"("string"=w285) -> ("trimmed string"=w175:string)  [unwired: 1 in]
  n249 = call <vilib>:"Trim Whitespace.vi"("string"=w284) -> ("trimmed string"=w174:string)  [unwired: 1 in]
  n250 = Number To Decimal String(number=w263) -> ()  [unwired: 1 in, 1 out]
  n251 = call <vilib>:"Trim Whitespace.vi"("string"=w190) -> ("trimmed string"=w176:string)  [unwired: 1 in]
  n252 = call <vilib>:"Trim Whitespace.vi"("string"=w189) -> ("trimmed string"=w177:string)  [unwired: 1 in]
  n253 = Number To Decimal String(number=w187) -> ()  [unwired: 1 in, 1 out]
  n254 = call <vilib>:"Simple Error Handler.vi"("error in (no error)"=w183) -> ()  [unwired: 1 in, 8 out]
  n255 = call <vilib>:"Simple Error Handler.vi"("error in (no error)"=w357) -> ()  [unwired: 1 in, 8 out]
  n256 = call <vilib>:"Simple Error Handler.vi"("error in (no error)"=w356) -> ()  [unwired: 1 in, 8 out]
  n257 = Build Array(w176, w177, w175, w174) -> (w173:string[])
  n258 = Move(source path=w361, error in=w363, 10:"Target Path") -> (error out=w362:errorcluster)  [unwired: 2 in, 2 out]
  n259 = TDMS Set Properties(5:w173, 7:string[] ["PupilCam_DroppedFrameIndex", "PupilCam_NumberDropped", "WhiskCam_DroppedFrameIndex", "WhiskCam_NumberDropped"] ("channel name(s) in (Untitled)"), 8:w37, 11:w34) -> (0:w291:errorcluster, 3:w290:refnum<k34>)  [unwired: 2 in, 2 out]
  n260 = TDMS Close(8:w291, 11:w290) -> (0:w364:errorcluster, 3:w353:path)
  n261 = Path To String(path=w353) -> (string=w355:string)
  n262 = call <vilib>:"Simple Error Handler.vi"("error in (no error)"=w362) -> ()  [unwired: 1 in, 8 out]
  n263 = TDMS Defragment(4:w364, 7:w353) -> (0:w350:errorcluster)
  n264 = Concatenate Strings(w355, "_index" ("string")) -> (w352:string)
  n265 = String To Path(string=w352) -> (path=w351:path)
  n266 = Move(source path=w353, error in=w350, 10:"Target Path") -> (error out=w358:errorcluster)  [unwired: 2 in, 2 out]
  n267 = Move(source path=w351, error in=w350, 10:"Target Path") -> (error out=w184:errorcluster)  [unwired: 2 in, 2 out]
  n268 = call <vilib>:"Simple Error Handler.vi"("error in (no error)"=w358) -> ()  [unwired: 1 in, 8 out]
  n269 = call <vilib>:"Simple Error Handler.vi"("error in (no error)"=w184) -> ()  [unwired: 1 in, 8 out]
